vi "LSP050Circuit.vi"(11 "water_level":dbl) -> (3 "voltage":dbl)   [LabVIEW 2020]
doc: "Simulates the conversion of liquid level in the tank to voltage as done by the LSP050 with the conditioning circuit. Considers the input water_level is already the delayed response."
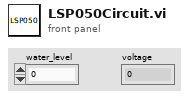
[diagram p1: front panel]
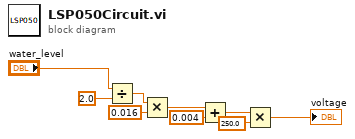
[diagram p0: block diagram]
diagram:
  n1 = Divide(x="water_level", y=2.0) -> (x/y=w3:dbl)
  n2 = Multiply(x=w3, y=0.016) -> (x*y=w5:dbl)
  n3 = Add(x=w5, y=0.004) -> (x+y=w7:dbl)
  n4 = Multiply(x=w7, y=250.0) -> (x*y=→"voltage":dbl)
